vi "Post Core.vi"(8 "error in (no error)":errorcluster, 11 "Simple Actor in":refnum<class "Simple Actor.lvclass">) -> (0 "error out":errorcluster, 3 "Simple Actor out":refnum<class "Simple Actor.lvclass">)   [LabVIEW 2020, in "Simple Actor.lvlib" / "Simple Actor.lvclass"]
uses:
  Simple Actor.lvclass
  Simple Actor.lvclass/Simple Actor.ctl
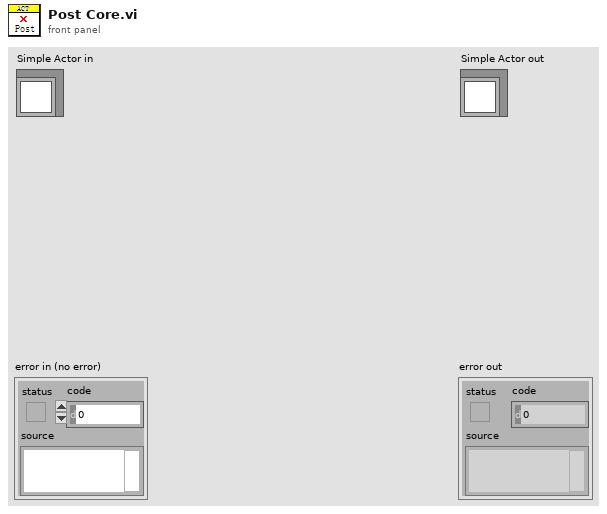
[diagram p1: front panel]
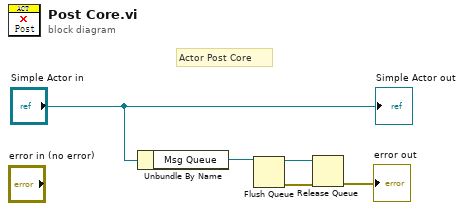
[diagram p0: block diagram]
diagram:
  # "Actor Post Core"
  n1 = Unbundle By Name("Simple Actor in") -> ("Msg Queue"=w4:refnum<queue>)
  n2 = Flush Queue(queue=w4) -> (queue out=w3:refnum<queue>, error out=w2:errorcluster)  [unwired: 1 in, 1 out]
  n3 = Release Queue(queue=w3, error in (no error)=w2) -> (error out=→"error out":errorcluster)  [unwired: 1 in, 2 out]
  "Simple Actor out" <- "Simple Actor in"
